vi "Channels Configuration Topology Data.vi"(8 "error in (no error)":errorcluster, 10 "Topology":string(combo)="2503/2-Wire 24x1 Mux") -> (0 "error out":errorcluster, 2 "Topology Data":T1)   [LabVIEW 2015]
uses:
  Configuration Controls/Topology Data.ctl
  DMM-SWITCH-ScanList System Explorer.lvlib
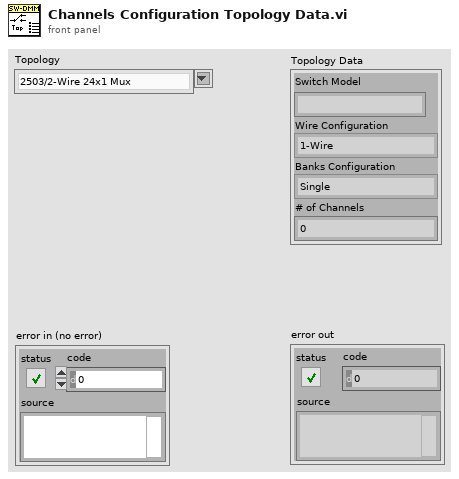
[diagram p1: front panel]
types:
  T1 = typedef "DMM-SWITCH-ScanList System Explorer.lvlib/Topology Data.ctl" = cluster{"Switch Model":string, "Wire Configuration":enum16{"1-Wire", "2-Wire", "4-Wire"}, "Banks Configuration":enum16{"Single", "Dual", "Quad", "Octal", "Sixteen"}, "# of Channels":u32}
  T2 = enum16{"Single", "Dual", "Quad", "Octal", "Sixteen"}
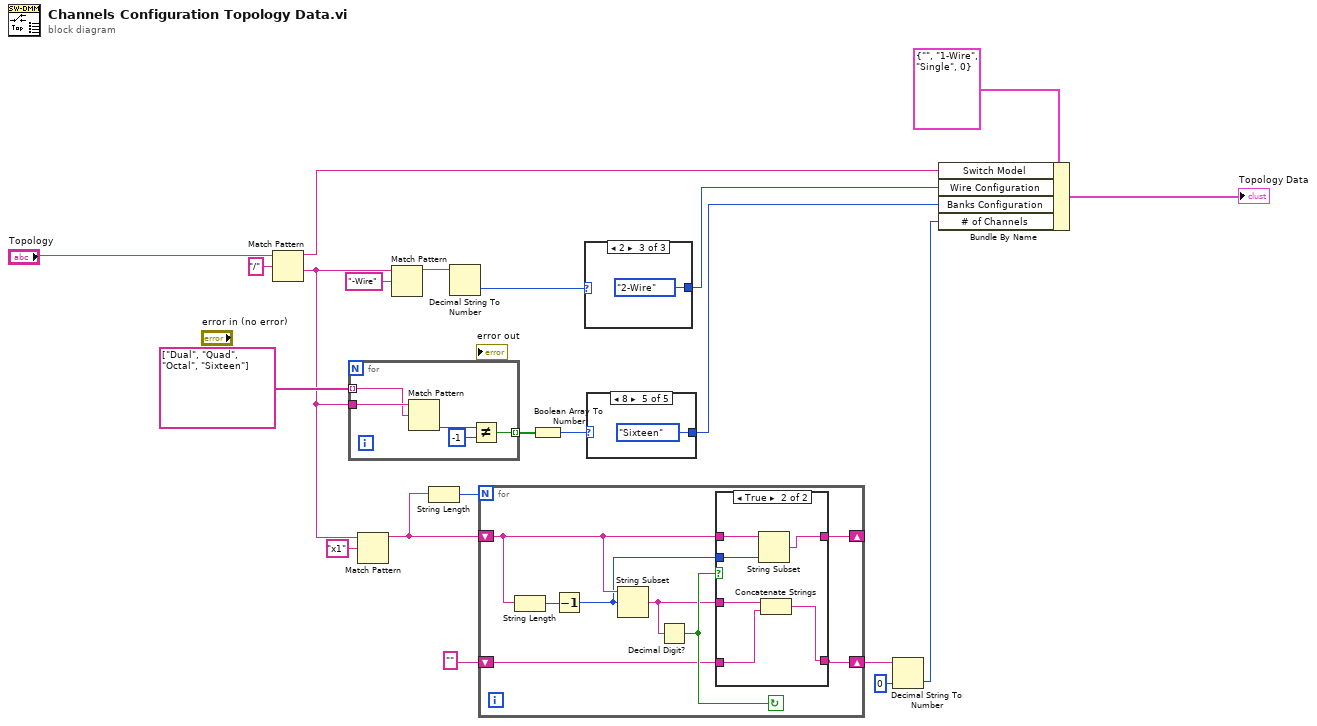
[diagram p0: block diagram]
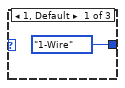
[diagram p2: hidden frame]
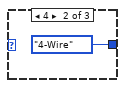
[diagram p3: hidden frame]
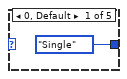
[diagram p5: hidden frame]
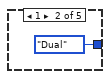
[diagram p6: hidden frame]
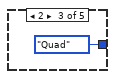
[diagram p7: hidden frame]
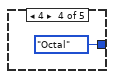
[diagram p8: hidden frame]
diagram:
  n1 = Match Pattern(string="Topology", regular expression="/") -> (before substring=w10:string, after substring=w7:string)  [unwired: 1 in, 2 out]
  n2 = for {
    tunnel: string[] ["Dual", "Quad", "Octal", "Sixteen"] ("Array") -> [w23] mode=indexing
    tunnel: w7 -> [w24]
    tunnel: [w22] -> w17 mode=indexing
    n3 = Match Pattern(string=w24, regular expression=w23) -> (offset past match=w25:i32)  [unwired: 1 in, 3 out]
    n4 = Not Equal?(x=w25, y=-1) -> (x != y?=w22:bool)
  }
  n5 = Match Pattern(string=w7, regular expression="x1") -> (before substring=w8:string)  [unwired: 1 in, 3 out]
  n6 = Match Pattern(string=w7, regular expression="-Wire") -> (before substring=w6:string)  [unwired: 1 in, 3 out]
  n7 = String Length(string=w8) -> (length=w12:i32)
  n8 = Decimal String To Number(string=w6) -> (number=w5:i32)  [unwired: 2 in, 1 out]
  n9 = for {
    N: w12 -> [_]
    shift-right: [w31] -> _
    shift-left: w8 -> [w33]
    shift-right: [w27] -> w3
    shift-left: "" -> [w29]
    stop <- w30 continue-if-true
    n10 = String Length(string=w33) -> (length=w34:i32)
    n11 = Decrement(x=w34) -> (x-1=w32:i32)
    n12 = String Subset(string=w33, offset (0)=w32) -> (substring=w28:string)  [unwired: 1 in]
    n13 = Decimal Digit?(1:w28) -> (0:w30:bool)
    n14 = case shown="True" w30 {
      tunnel: w33 -> [w36 w42]
      tunnel: w32 -> [_ w40]
      tunnel: [w36 w41] -> w31
      tunnel: w29 -> [w35 w37]
      tunnel: w28 -> [_ w38]
      tunnel: [w35 w39] -> w27
      frame False {
      }
      frame True {
        n15 = String Subset(string=w42, length (rest)=w40) -> (substring=w41:string)  [unwired: 1 in]
        n16 = Concatenate Strings(w38, w37) -> (w39:string)
      }
    }
  }
  n17 = Boolean Array To Number(Boolean array=w17) -> (number=w16:u32)
  n18 = case shown="2" w5 {
    tunnel: [enum16{"1-Wire", "2-Wire", "4-Wire"}."1-Wire" ("Wire Configuration") enum16{"1-Wire", "2-Wire", "4-Wire"}."4-Wire" ("Wire Configuration") enum16{"1-Wire", "2-Wire", "4-Wire"}."2-Wire" ("Wire Configuration")] -> w4
    frame 1, Default {
    }
    frame 4 {
    }
    frame 2 {
    }
  }
  n19 = case shown="8" w16 {
    tunnel: [T2."Single" ("Banks Configuration") T2."Dual" ("Banks Configuration") T2."Quad" ("Banks Configuration") T2."Octal" ("Banks Configuration") T2."Sixteen" ("Banks Configuration")] -> w15
    frame 0, Default {
    }
    frame 1 {
    }
    frame 2 {
    }
    frame 4 {
    }
    frame 8 {
    }
  }
  n20 = Decimal String To Number(string=w3, default (0L)=u32 0 ("default (0 I32)")) -> (number=w2:u32)  [unwired: 1 in, 1 out]
  n21 = Bundle By Name(cluster=T1 {"Switch Model"="", "Wire Configuration"=enum."1-Wire", "Banks Configuration"=enum."Single", "# of Channels"=0} ("Topology Data"), "Switch Model"=w10, "Wire Configuration"=w4, "Banks Configuration"=w15, "# of Channels"=w2) -> (→"Topology Data":T1)
